vi "Create Stream State Register.vi"() -> (3 "stream state register":T1)   [LabVIEW 2015, in "niInstr Streaming v1 FPGA.lvlib"]
doc: "Create resources necessary to handshake the stream.state indicator to a another loop.\n\nUse with Get/Set Stream State Register.vi"
uses:
  <instrlib>/_niInstr/Streaming/v1/FPGA/niInstr Streaming v1 FPGA.lvlib
  <instrlib>/_niInstr/Streaming/v1/FPGA/Public/Stream State Register.ctl
  <vilib>/rvi/DataTransferAndStorage/Container/Common/niFpgaContainerGetUniqueNameForEmu.vi
  <vilib>/rvi/DataTransferAndStorage/Container/Common/niFpgaContainerSetEmuInfo.vi
  <vilib>/rvi/eio/common/nirviEmuReportErrorAndStop.vi
  <vilib>/rvi/LocalResourceManager/LocalResourceManager.xnode
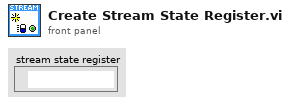
[diagram p1: front panel]
types:
  T1 = typedef "niInstr Streaming v1 FPGA.lvlib/Stream State Register.ctl" = refnum<k21>
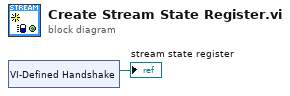
[diagram p0: block diagram]
diagram:
  n1 = xnode "VI-Defined Handshake"() -> ("Handshake Out"=→"stream state register":refnum<k21>)
